vi "左启动全局.vi"() -> ()   [LabVIEW 2014]
panel:
  in  "左启动":bool
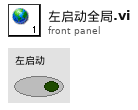
[diagram p1: front panel]
diagram:
